vi "Write Step Data(DC Manual).vi"(7 "Mem Number":u32=1 min=1 max=50, 8 "Error In":errorcluster, 9 "AC Advance Step Data":T1 {"Transient Time" format="%.1f ms"; "Transient Site" format="%.0f ¢X"; "Transient Volt" format="%.1f V"; "CF Lo Limit" format="%.2f"; "CF Hi Limit" format="%.2f"; "Q Lo Limit" format="%.0f VAR"; "Q Hi Limit" format="%.0f VAR"; "VA Lo Limit" format="%.0f VA"; "VA Hi Limit" format="%.0f VA"; "PF Lo Limit" format="%.3f"; "PF Hi Limit" format="%.3f"; "P Lo Limit" format="%.0f W"; "P Hi Limit" format="%.0f W"; "AP Lo Limit" format="%.1f A"; "AP Hi Limit" format="%.1f A"; "A Lo Limit" format="%.2f A"; "A Hi Limit" format="%.2f A"; "Delay Time" format="%.1f s"; "£GT" format="%.0f ms"; "£GF" format="%.1f Hz"; "£GV" format="%.1f V"; "Time" format="%.1f s"; "Voltage" format="%.1f V"; "Frequency" format="%.1f Hz"}, 10 "Modbus ID":string, 11 "VISA resource name":refnum<visa-resource-name>) -> (0 "Error Out":errorcluster, 3 "VISA resource name out":refnum<visa-resource-name>)   [LabVIEW 2013]
uses:
  Utility/Get Step Address(DC Manual).vi
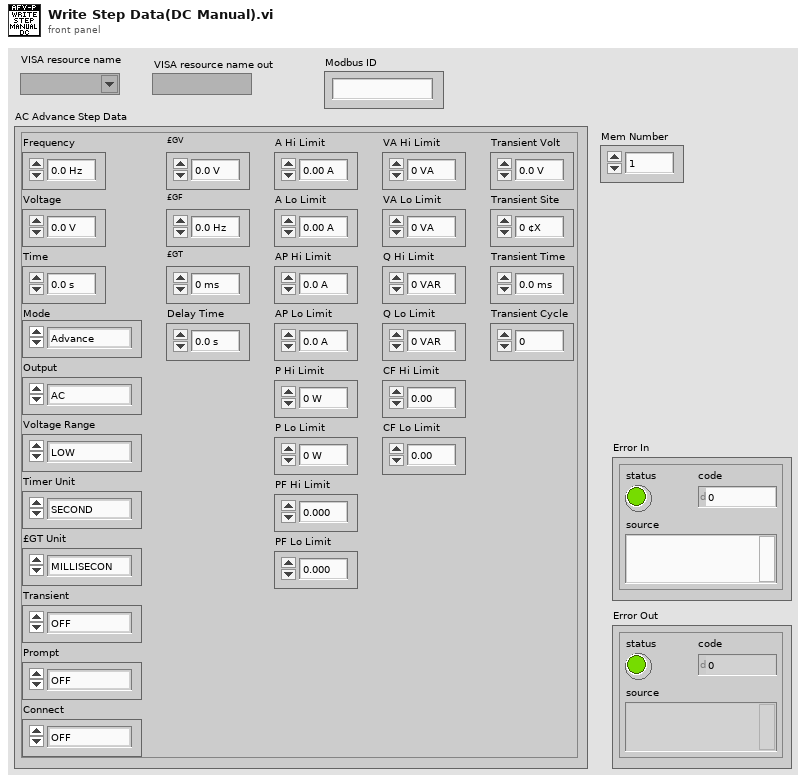
[diagram p1: front panel]
types:
  T1 = cluster{"Frequency":dbl, "Voltage":dbl, "Time":dbl, "Mode":enum16{"Advance", "Basic"}, "Output":enum16{"AC", "DC"}, "Voltage Range":enum16{"LOW", "HIGH", "AUTO"}, "Timer Unit":enum16{"SECOND", "MINUTE", "HOUR"}, "£GT Unit":enum16{"MILLISECON", "SECOND", "CYCLE"}, "Transient":enum16{"OFF", "ON"}, "Prompt":enum16{"OFF", "ON"}, "Connect":enum16{"OFF", "ON"}, "£GV":dbl, "£GF":dbl, "£GT":u16, "Delay Time":dbl, "A Hi Limit":dbl, "A Lo Limit":dbl, "AP Hi Limit":dbl, "AP Lo Limit":dbl, "P Hi Limit":u16, "P Lo Limit":u16, "PF Hi Limit":dbl, "PF Lo Limit":dbl, "VA Hi Limit":u16, "VA Lo Limit":u16, "Q Hi Limit":u16, "Q Lo Limit":u16, "CF Hi Limit":dbl, "CF Lo Limit":dbl, "Transient Volt":dbl, "Transient Site":u16, "Transient Time":dbl, "Transient Cycle":u16}
  T2 = cluster{"ID":string, "Function Code":string, "Length (High)":string, "Length (Low)":string, "Start Address (High)":string, "Start Address (Middle High)":string, "Start Address (Middle Low)":string, "Start Address (Low)":string, "Data":string}
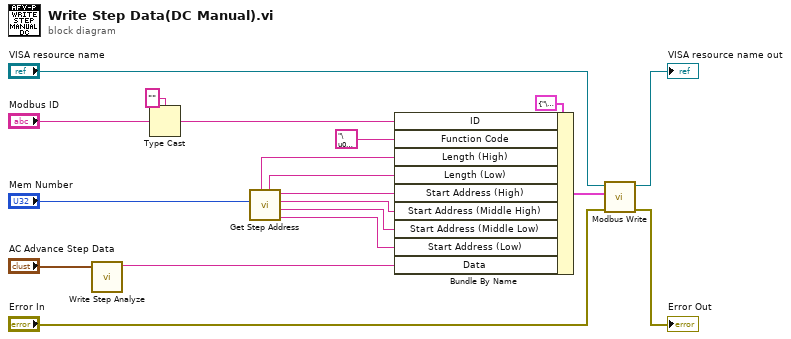
[diagram p0: block diagram]
diagram:
  n1 = call "Write Step Analyze.vi"("AC Advance Step Data"="AC Advance Step Data") -> ("Data"=w11:string)  [unwired: 10 in]
  n2 = Type Cast(type="" ("Binary Data (Hex) 3"), x="Modbus ID") -> (*(type *) &x=w8:string)
  n3 = call-poly "Get Step Address.vi"("Program Data.Mem Number"="Mem Number") -> ("Program Data.Start Address (Low)"=w2:string, "Program Data.Start Address (Middle Low)"=w3:string, "Program Data.Start Address (Middle High)"=w4:string, "Program Data.Start Address (High)"=w7:string, "Length (Low)"=w6:string, "Length (High)"=w5:string)  [unwired: 5 in]
  n4 = Bundle By Name(cluster=T2 {"ID"="\u0000", "Function Code"="\u0000", "Length (High)"="\u0000", "Length (Low)"="\u0000", "Start Address (High)"="\u0000", "Start Address (Middle High)"="\u0000", "Start Address (Middle Low)"="\u0000", "Start Address (Low)"="\u0000", "Data"=""} ("Write Buffer"), "ID"=w8, "Function Code"="\u0010", "Length (High)"=w5, "Length (Low)"=w6, "Start Address (High)"=w7, "Start Address (Middle High)"=w4, "Start Address (Middle Low)"=w3, "Start Address (Low)"=w2, "Data"=w11) -> (w15:T2)
  n5 = call "Modbus Write.vi"("Error In"="Error In", "Write Buffer"=w15, "VISA resource name"="VISA resource name") -> ("Error Out"=→"Error Out":errorcluster, "VISA resource name out"=→"VISA resource name out":refnum<visa-resource-name>)  [unwired: 7 in]
